vi "Overview Cursor Move.vi"(8 "error in":errorcluster, 11 "XYGraphOverview in":refnum<class "XYGraphOverview.lvclass">) -> (0 "error out":errorcluster, 3 "XYGraphOverview out":refnum<class "XYGraphOverview.lvclass">)   [LabVIEW 2020, in "XYGraphOverview.lvlib" / "XYGraphOverview.lvclass"]
uses:
  XYGraphOverview.lvclass
  XYGraphOverview.lvclass/XYGraphOverview.ctl
  Read Highlight Block Color.vi
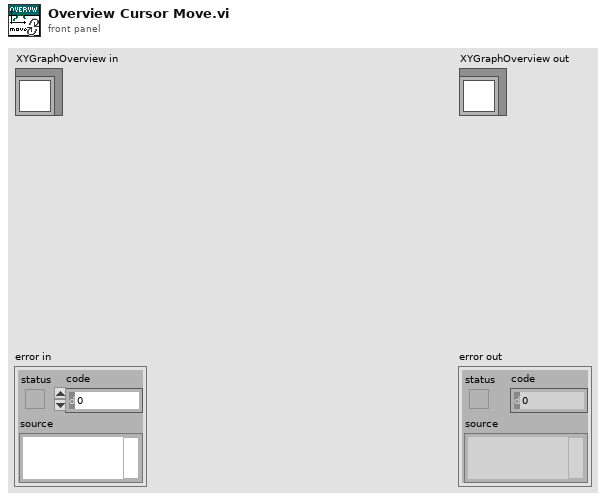
[diagram p1: front panel]
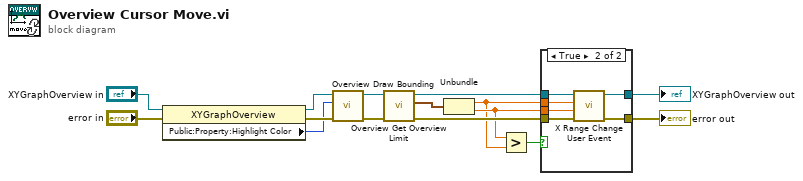
[diagram p0: block diagram]
diagram:
  n1 = property class="XYGraphOverview"(reference="XYGraphOverview in", error in="error in") -> (reference out=w5:refnum<class "XYGraphOverview.lvclass">, error out=w6:errorcluster, "Public:Property:Highlight Color"=w4:u32)
  n2 = call "Overview Draw Bounding.vi"("error in (no error)"=w6, "Color"=w4, "XYGraphOverview in"=w5) -> ("error out"=w15:errorcluster, "XYGraphOverview out"=w14:refnum<class "XYGraphOverview.lvclass">)  [unwired: 7 in]
  n3 = call "Overview Get Overview Limit.vi"("error in"=w15, "XYGraphOverview in"=w14) -> ("error out"=w11:errorcluster, "Limit"=w13:cluster{"Lower Limit":dbl, "Upper Limit":dbl}, "XYGraphOverview out"=w12:refnum<class "XYGraphOverview.lvclass">)  [unwired: 7 in]
  n4 = Unbundle(w13) -> ("Lower Limit"=w2:dbl, "Upper Limit"=w3:dbl)
  n5 = Greater?(x=w3, y=w2) -> (0:w1:bool)
  n6 = case shown="True" w1 {
    tunnel: w12 -> [w17 w23]
    tunnel: w11 -> [w16 w22]
    tunnel: [w17 w21] -> w10
    tunnel: [w16 w20] -> w9
    tunnel: w3 -> [_ w19]
    tunnel: w2 -> [_ w18]
    frame False {
    }
    frame True {
      n7 = call "X Range Change User Event.vi"("error in (no error)"=w22, "Upper Range"=w19, "Lower Range"=w18, "XYGraphOverview in"=w23) -> ("error out"=w20:errorcluster, "XYGraphOverview out"=w21:refnum<class "XYGraphOverview.lvclass">)  [unwired: 6 in]
    }
  }
  "error out" <- w9
  "XYGraphOverview out" <- w10
